vi "serial term1.vi"() -> ()   [LabVIEW 2015]
uses:
  <vilib>/Rock Robotics/WPI/SerialPort/WPI_SerialPort.ctl
panel:
  out "concatenated string":string
  in  "Continue":bool
  in  "Buffer":string
  out "error out":errorcluster
  in  "error in (no error)":errorcluster
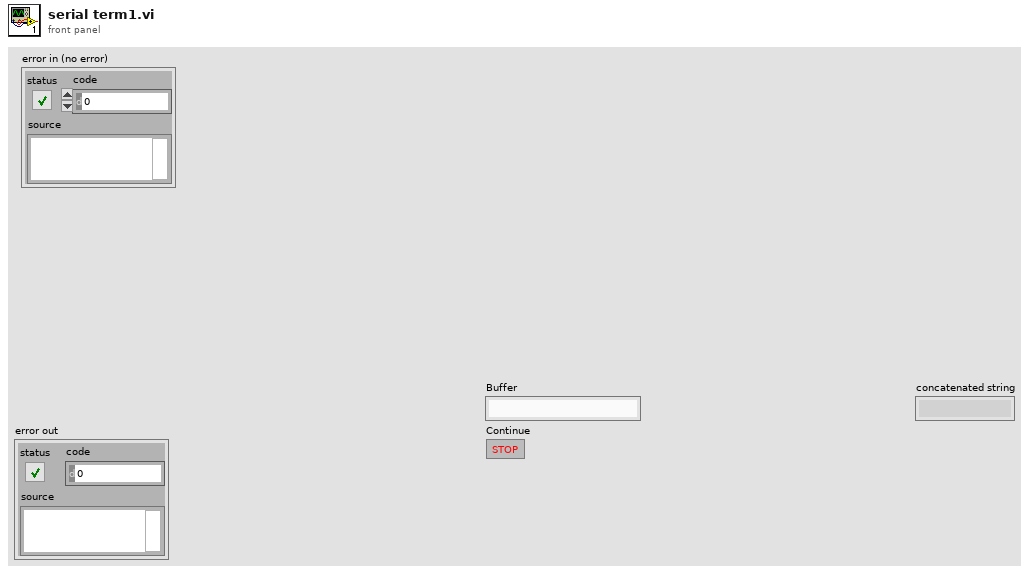
[diagram p1: front panel]
types:
  T1 = typedef "WPI_SerialPort.ctl" = enum16{"Onboard RS-232", "MXP TTL"}
  T2 = typedef "WPI_SerialPortRef.ctl" = cluster{"DevStatus":errorcluster, "Serial Port Name":refnum<visa-resource-name>}
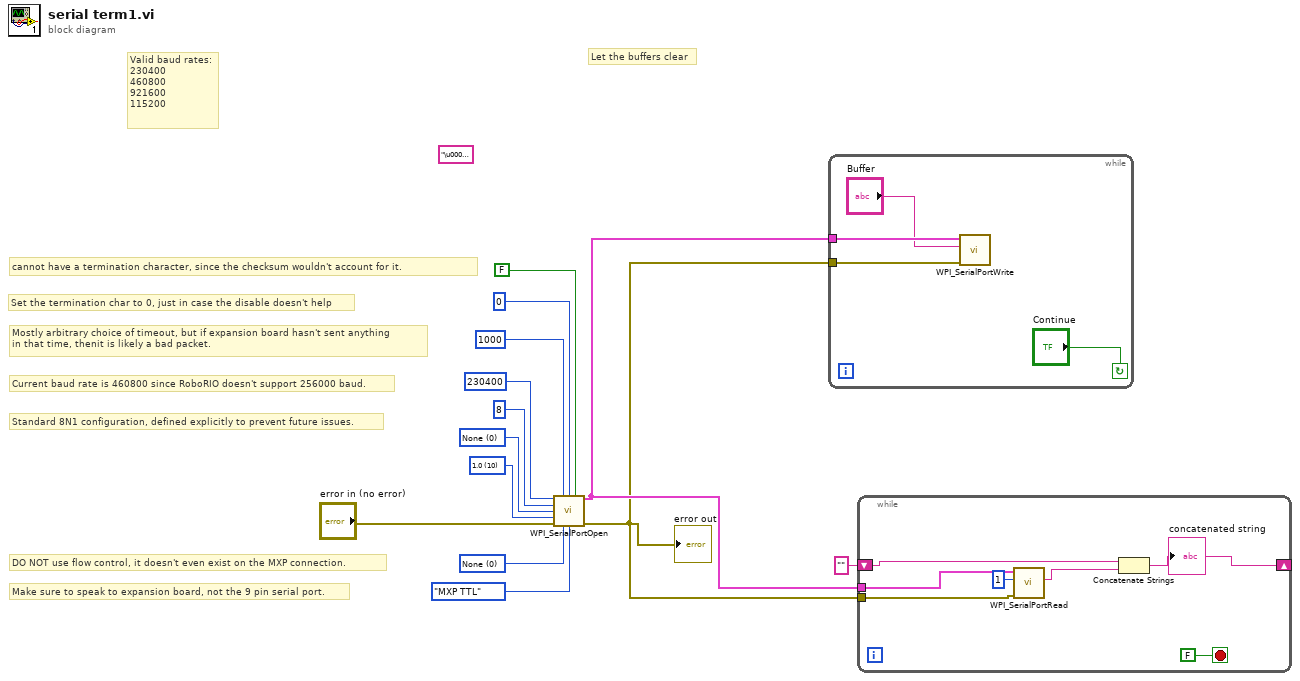
[diagram p0: block diagram]
diagram:
  (unwired) "\u0004\u0004" ("Buffer")
  w12 = u16 10 items=["1.0"=10, "1.5"=15, "2.0"=20] ("Stop Bits")
  w8 = u16 0 items=["None", "XON/XOFF", "RTS/CTS", "XON/XOFF & RTS/CTS", "DTR/DSR", "XON/XOFF & DTR/DSR"] ("Flow Control")
  w7 = u16 0 items=["None", "Odd", "Even", "Mark", "Space"] ("Parity")
  # "Let the buffers clear"
  # "Valid baud rates:\n230400\n460800\n921600\n115200"
  # "Make sure to speak to expansion board, not the 9 pin serial port."
  # "DO NOT use flow control, it doesn't even exist on the MXP connection."
  # "Standard 8N1 configuration, defined explicitly to prevent future issues."
  # "Current baud rate is 460800 since RoboRIO doesn't support 256000 baud."
  # "Mostly arbitrary choice of timeout, but if expansion board hasn't sent anything\nin that time, thenit is likely a bad packet."
  # "Set the termination char to 0, just in case the disable doesn't help"
  # "cannot have a termination character, since the checksum wouldn't account for it."
  n1 = call <vilib>:"WPI_SerialPortOpen.vi"("Baud Rate"=u32 230400, "Timeout Value (ms)"=u32 1000, "Termination Char (0xA = '\\n' = LF)"=u8 0 ("Termination Char (0xA = '\\n' = LF)"), "Enable Termination Char? (T)"=FALSE, "Data Bits"=u16 8, "Parity"=w7, "Stop Bits"=w12, "error in (no error)"="error in (no error)", "Flow Control"=w8, "Serial Port"=WPI_SerialPort."MXP TTL") -> ("SerialPortRef"=w3:T2, "error out"=w1:errorcluster)  [unwired: 4 in]
  "error out" <- w1
  n2 = while {
    tunnel: w3 -> [w17]
    tunnel: w1 -> [w16]
    stop <- "Continue" continue-if-true
    n3 = call <vilib>:"WPI_SerialPortWrite.vi"("error in (no error)"=w16, "Buffer"="Buffer", "SerialPortRef"=w17) -> ()  [unwired: 6 in, 3 out]
  }
  n4 = while {
    tunnel: w3 -> [w24]
    shift-right: [w22] -> _
    shift-left: "" -> [w21]
    tunnel: w1 -> [w20]
    stop <- FALSE stop-if-true
    n5 = call <vilib>:"WPI_SerialPortRead.vi"("error in (no error)"=w20, "Num Bytes to Read"=u32 1, "SerialPortRef"=w24) -> ("Buffer"=w23:string)  [unwired: 6 in, 2 out]
    n6 = Concatenate Strings(w21, w23) -> (w22:string)
    "concatenated string" <- w22
  }
